vi "Get_TargetFile_Destination_Paths.vi"(8 "error in (no error)":errorcluster, 11 "AB_Targetfile in":refnum<class "AB_Targetfile.lvclass">) -> (0 "error out":errorcluster, 1 "support path":path, 2 "destination path":path, 3 "AB_Targetfile out":refnum<class "AB_Targetfile.lvclass">, 4 "targetfile path":path)   [LabVIEW 2020, in "AB_Targetfile.lvclass"]
uses:
  <vilib>/AppBuilder/AB_Classes/TargetFile/AB_Targetfile.lvclass
  e:/builds/penguin/labview/branches/2020/dev/dist/vi.lib/AppBuilder/AB_Classes/Build/AB_Build.lvclass
  <vilib>/AppBuilder/AB_Classes/Destination/AB_Destination.lvclass
  <vilib>/AppBuilder/AB_Classes/Build/AB_Build.lvclass
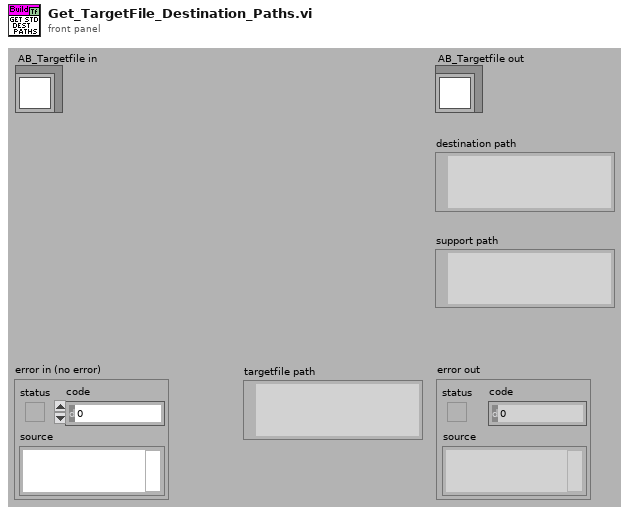
[diagram p1: front panel]
types:
  T1 = typedef "AB_Build.ctl" = cluster{"buildSpecName":string, "buildSpecDescription":string, "destinations":refnum<class "AB_Destination.lvclass">[], "exclusionOption":T2, "defaultLanguage":string, "supportedLanguages":string[], "excludedDirectories":path[], "buildContext":refnum<vi>, "buildObject":T3, "preview":bool, "programatic":bool, "progressBarEvents":T4, "userLog_Path":path, "preActionID":string, "preAction_Path":path, "postActionID":string, "postAction_Path":path, "eng_checkForBrokenVIs?":bool, "eng_verboseLinkerErrors?":bool, "localDest_Path":path, "targetDest_Path":path, "removeVIObject":u16, "cache":refnum<class "PreviewCache.lvclass">, "use cache":bool, "previewCache_ID":string, "buildCache_ID":string, "eng_TempLocalDest_Path":path, "eng_collectDependencies?":bool, "versionInfo":cluster{"buildVersion":cluster{"major":u16, "minor":u16, "patch":u16, "build":u16}, "autoIncrement":bool}, "eng_enableVIChecksums":bool}
  T2 = typedef "AB_Exclusion_Option.ctl" = cluster{"typedefs":bool, "polymorphicVIs":bool, "unusedLibraryItems":bool, "modifyLibraryFile":bool, "edit-timeDependencies":bool, "inlineVIs":bool, "dependent PPLs":bool, "dependent DLLs":bool}
  T3 = typedef "ItemRef.ctl" = u64
  T4 = typedef "provcom_ProgressBar_Events.ctl" = cluster{"newJob":refnum<user-event>, "newItem":refnum<user-event>, "errorMsg":T5, "cancel":refnum<user-event>}
  T5 = typedef "mxLvBuildError.ctl" = refnum<user-event>
  T6 = typedef "AB_Destination.ctl" = cluster{"destName":string, "path":path, "libraryName":string, "preserveHierarchy":bool, "eng_inBuild":bool, "eng_libraryReference":refnum<vi>, "eng_restictAddToNewLibrary":bool}
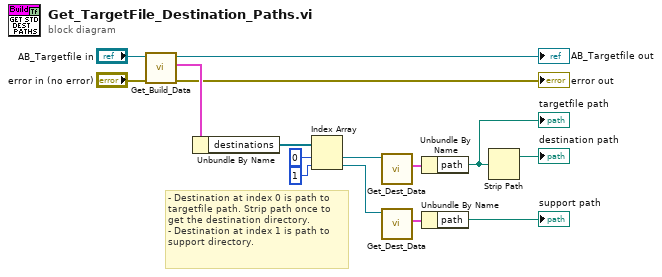
[diagram p0: block diagram]
diagram:
  # "- Destination at index 0 is path to targetfile path. Strip path once to get the destination directory.\n- Destination at index 1 is path to support directory."
  n1 = call <vilib>:"Get_Build_Data.vi"("error in (no error)"="error in (no error)", "Class in"="AB_Targetfile in") -> ("error out"=→"error out":errorcluster, "data"=w7:T1, "Class out"=→"AB_Targetfile out":refnum<class "AB_Targetfile.lvclass">)  [unwired: 7 in]
  n2 = Unbundle By Name(w7) -> ("destinations"=w6:refnum<class "AB_Destination.lvclass">[])
  n3 = Index Array(array=w6, index #1=0 ("index"), index #2=1 ("index")) -> (element #1=w13:refnum<class "AB_Destination.lvclass">, element #2=w10:refnum<class "AB_Destination.lvclass">)
  n4 = call <vilib>:"Get_Dest_Data.vi"("Class in"=w13) -> ("destName"=w14:T6)  [unwired: 8 in, 2 out]
  n5 = call <vilib>:"Get_Dest_Data.vi"("Class in"=w10) -> ("destName"=w11:T6)  [unwired: 8 in, 2 out]
  n6 = Unbundle By Name(w14) -> ("path"=w1:path)
  "targetfile path" <- w1
  n7 = Unbundle By Name(w11) -> ("path"=→"support path":path)
  n8 = Strip Path(path=w1) -> (stripped path=→"destination path":path)  [unwired: 1 out]
